vi "Initialize.vi"() -> (14 "Fatal Error Out":T11, 15 "State Out":T1)   [LabVIEW 2021, in "myRIO AI Continuous Open.xnode"]
uses:
  <vilib>/myRIO/Instrument Drivers/Onboard IO/AI Continuous/vis/myRIO AI Continuous Open.xnode
  <vilib>/XNodeSupport/XNodeErrorCluster.ctl
  <vilib>/myRIO/Instrument Drivers/Onboard IO/AI Continuous/vis/State.ctl
  <vilib>/myRIO/Common/Instrument Driver Framework/Utilities/typedefs/myRIOXPeripheral.ctl
  <vilib>/XNodeSupport/XNodeTerm4Array.ctl
  <vilib>/XNodeSupport/XNodeTerm4.ctl
  <vilib>/XNodeSupport/XNodeString.ctl
  <vilib>/XNodeSupport/XNodeVariant.ctl
  <vilib>/XNodeSupport/XNodeRect32.ctl
  <vilib>/XNodeSupport/XNodeInt.ctl
  <vilib>/XNodeSupport/XNodeBool.ctl
  <vilib>/XNodeSupport/XNodeTermDirection.ctl
  <vilib>/myRIO/Instrument Drivers/Onboard IO/AI Continuous/typedefs/AI Continuous Reference.ctl
  <vilib>/myRIO/Common/Instrument Driver Framework/Utilities/typedefs/myRIO Generic Hardware Reference.ctl
  <vilib>/myRIO/Common/Instrument Driver Framework/Utilities/typedefs/Hardware Version Enum.ctl
  <vilib>/myRIO/Common/Instrument Driver Framework/Utilities/typedefs/myRIO v1.0 Reference.ctl
  <vilib>/myRIO/Common/Instrument Driver Framework/Utilities/typedefs/Generic FPGA Reference.ctl
  <vilib>/myRIO/Common/Instrument Driver Framework/ELVIS III v1.0/AI Continuous/typedefs/AI Continuous Channels List.ctl
  <vilib>/myRIO/Common/Instrument Driver Framework/ELVIS III v1.0/AI Continuous/typedefs/ELVIS III v1.0 AI Continuous Channels Enum.ctl
  <vilib>/myRIO/Common/Instrument Driver Framework/Utilities/typedefs/Analog Scaling Constants.ctl
  <vilib>/myRIO/Instrument Drivers/Onboard IO/AO Block/vis/State.ctl
  <vilib>/myRIO/Common/Instrument Driver Framework/Utilities/vis/myRIOXGlobal.vi
  <vilib>/XNodeSupport/NI_XNodeSupport.lvlib
  <vilib>/myRIO/Instrument Drivers/Onboard IO/AO Block/vis/myRIO AO N Samples Open.xnode
  <vilib>/myRIO/Instrument Drivers/Onboard IO/AI Continuous/AI Continuous.lvlib
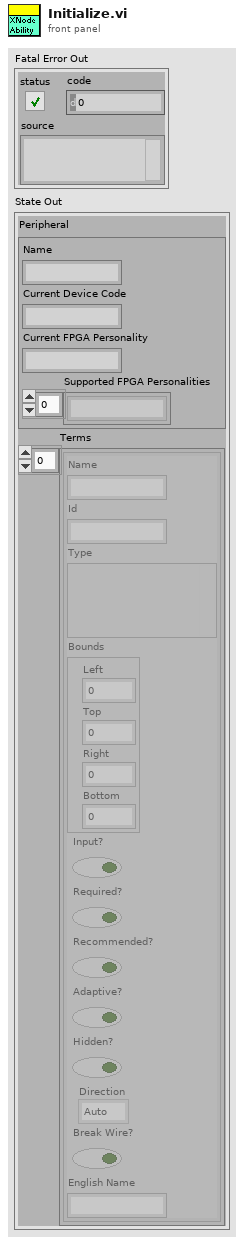
[diagram p1: front panel]
types:
  T1 = typedef "myRIO AI Continuous Open.xnode/State.ctl" = cluster{"Peripheral":T2, "Terms":T3}
  T2 = typedef "myRIOXPeripheral.ctl" = cluster{"Name":string, "Current Device Code":string, "Current FPGA Personality":string, "Supported FPGA Personalities":string[]}
  T3 = typedef "NI_XNodeSupport.lvlib/XNodeTerm4Array.ctl" = T4[]
  T4 = typedef "NI_XNodeSupport.lvlib/XNodeTerm4.ctl" = cluster{"Name":T5, "Id":T5, "Type":T6, "Bounds":T7, "Input?":T9, "Required?":T9, "Recommended?":T9, "Adaptive?":T9, "Hidden?":T9, "Direction":T10, "Break Wire?":T9, "English Name":T5}
  T5 = typedef "NI_XNodeSupport.lvlib/XNodeString.ctl" = string
  T6 = typedef "NI_XNodeSupport.lvlib/XNodeVariant.ctl" = variant
  T7 = typedef "NI_XNodeSupport.lvlib/XNodeRect32.ctl" = cluster{"Left":T8, "Top":T8, "Right":T8, "Bottom":T8}
  T8 = typedef "NI_XNodeSupport.lvlib/XNodeInt.ctl" = i32
  T9 = typedef "NI_XNodeSupport.lvlib/XNodeBool.ctl" = bool
  T10 = typedef "NI_XNodeSupport.lvlib/XNodeTermDirection.ctl" = enum32{"Auto", "Up", "Down", "Left", "Right", "Center"}
  T11 = typedef "NI_XNodeSupport.lvlib/XNodeErrorCluster.ctl" = errorcluster
  T12 = typedef "AI Continuous.lvlib/AI Continuous Reference.ctl" = cluster{"myRIO Reference":T13, "AI (Continuous) Channels List":T17, "AI (Continuous) Scaling Constants List":T19[], "Bank Count":u8[]}
  T13 = typedef "myRIO Generic Hardware Reference.ctl" = cluster{"myRIO Model":T14, "myRIO Hardware Reference":T15}
  T14 = typedef "Hardware Version Enum.ctl" = enum16{"Unknown", "myRIO-1900", "myRIO-1950", "roboRIO", "NI ELVIS RIO CM", "ELVIS III"}
  T15 = typedef "myRIO v1.0 Reference.ctl" = cluster{"Generic FPGA Reference":T16, "Allow multiple opens":bool}
  T16 = typedef "Generic FPGA Reference.ctl" = refnum<k20>
  T17 = typedef "AI Continuous Channels List.ctl" = T18[]
  T18 = typedef "ELVIS III v1.0 AI Continuous Channels Enum.ctl" = enum16{"Not Connected", "A/AI0 (Continuous)", "A/AI1 (Continuous)", "A/AI2 (Continuous)", "A/AI3 (Continuous)", "A/AI4 (Continuous)", "A/AI5 (Continuous)", "A/AI6 (Continuous)", "A/AI7 (Continuous)", "A/AI0 (DIFF Continuous)", "A/AI1 (DIFF Continuous)", "A/AI2 (DIFF Continuous)", "A/AI3 (DIFF Continuous)", "B/AI0 (Continuous)", "B/AI1 (Continuous)", "B/AI2 (Continuous)", "B/AI3 (Continuous)", "B/AI4 (Continuous)", "B/AI5 (Continuous)", "B/AI6 (Continuous)", "B/AI7 (Continuous)", "B/AI0 (DIFF Continuous)", "B/AI1 (DIFF Continuous)", "B/AI2 (DIFF Continuous)", "B/AI3 (DIFF Continuous)"}
  T19 = typedef "Analog Scaling Constants.ctl" = cluster{"LSB Weight (Volts)":dbl, "Offset (Volts)":dbl, "Signed?":bool}
  T20 = typedef "myRIO AO N Samples Open.xnode/State.ctl" = cluster{"Peripheral":T2, "Terms":T3}
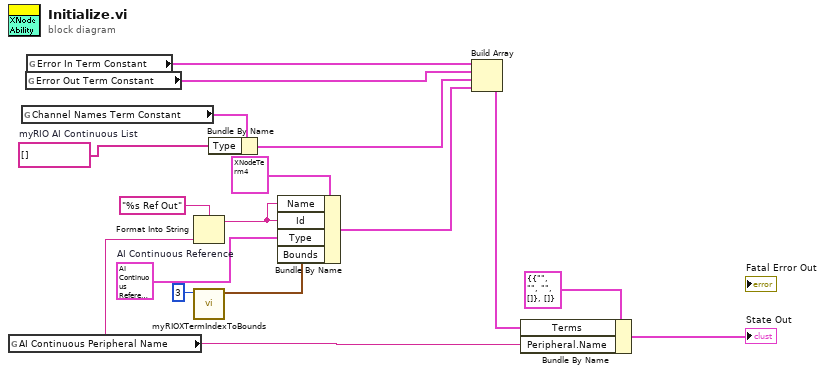
[diagram p0: block diagram]
diagram:
  w1 = tag[] []  # myRIO AI Continuous List
  w2 = T12 {"myRIO Reference"={"myRIO Model"=enum."Unknown", "myRIO Hardware Reference"={"Generic FPGA Reference"=refnum, "Allow multiple opens"=FALSE}}, "AI (Continuous) Channels List"=[], "AI (Continuous) Scaling Constants List"=[], "Bank Count"=[]}  # AI Continuous Reference
  n1 = global read "myRIOXGlobal.vi" "AI Continuous Peripheral Name"() -> (w5:string)
  n2 = global read "myRIOXGlobal.vi" "Channel Names Term Constant"() -> (w8:T4)
  n3 = global read "myRIOXGlobal.vi" "Error Out Term Constant"() -> (w14:T4)
  n4 = global read "myRIOXGlobal.vi" "Error In Term Constant"() -> (w15:T4)
  n5 = Format Into String(format string="%s Ref Out" ("Name"), w5) -> (resulting string=w12:string)  [unwired: 2 in, 1 out]
  n6 = call <vilib>:"myRIOXTermIndexToBounds.vi"("Index"=3) -> ("Bounds"=w11:T7)  [unwired: 10 in]
  n7 = Bundle By Name(cluster=w8, "Type"=w1) -> (w7:T4)
  n8 = Bundle By Name(cluster=T4 {"Name"="", "Id"="", "Type"=variant, "Bounds"={"Left"=0, "Top"=0, "Right"=0, "Bottom"=0}, "Input?"=FALSE, "Required?"=FALSE, "Recommended?"=TRUE, "Adaptive?"=FALSE, "Hidden?"=FALSE, "Direction"=enum."Auto", "Break Wire?"=FALSE, "English Name"=""} ("Channel Names Term Constant"), "Name"=w12, "Id"=w12, "Type"=w2, "Bounds"=w11) -> (w6:T4)
  n9 = Build Array(w15, w14, w7, w6) -> (w4:T4[])
  n10 = Bundle By Name(cluster=T20 {"Peripheral"={"Name"="", "Current Device Code"="", "Current FPGA Personality"="", "Supported FPGA Personalities"=[]}, "Terms"=[]} ("State Out"), "Terms"=w4, "Peripheral.Name"=w5) -> (→"State Out":T20)
